vi "Sparse Signal FFT.vi"(2 "signal length":i32=1, 3 "X":cdb[](array[numeric]) format="%.2f") -> (0 "error":i32, 1 "FFT {X}":cdb[](array[numeric]) format="%.2f")   [LabVIEW 2020, in "NI_Gmath.lvlib"]
doc: "Computes the Fourier transform of sparse signals faster than the FFT does."
uses:
  <vilib>/gmath/NI_Gmath.lvlib
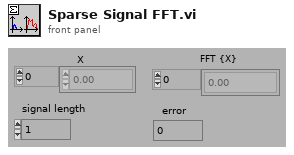
[diagram p1: front panel]
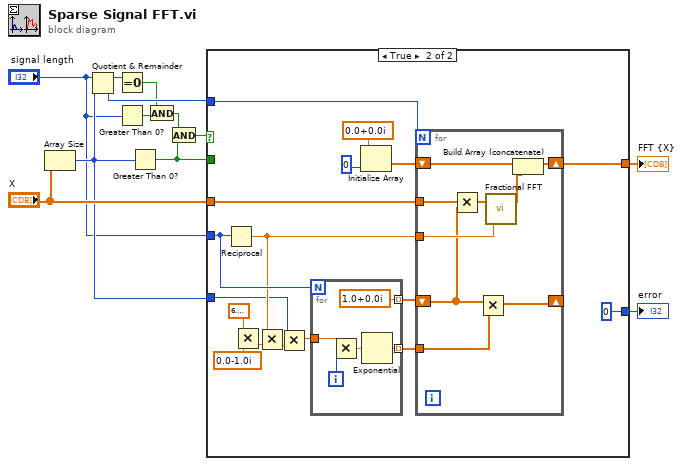
[diagram p0: block diagram]
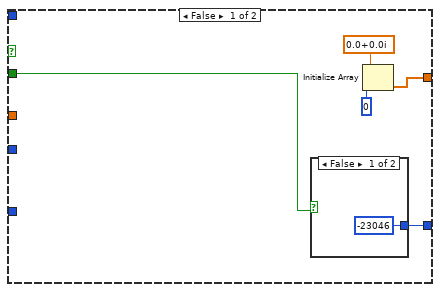
[diagram p2: hidden frame]
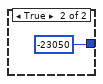
[diagram p3: hidden frame]
diagram:
  n1 = Array Size(array="X") -> (size(s)=w5:i32)
  n2 = Quotient & Remainder(x="signal length", y=w5) -> (x-y*floor(x/y)=w11:i32, floor(x/y)=w9:i32)
  n3 = Equal To 0?(x=w11) -> (x = 0?=w2:bool)
  n4 = Greater Than 0?(x="signal length") -> (x > 0?=w3:bool)
  n5 = Greater Than 0?(x=w5) -> (x > 0?=w8:bool)
  n6 = And(x=w2, y=w3) -> (x .and. y?=w1:bool)
  n7 = And(x=w1, y=w8) -> (x .and. y?=w10:bool)
  n8 = case shown="True" w10 {
    tunnel: "X" -> [_ w35]
    tunnel: [w15 w31] -> w7
    tunnel: [w13 0] -> w12
    tunnel: w8 -> [w14 _]
    tunnel: "signal length" -> [_ w25]
    tunnel: w9 -> [_ w21]
    tunnel: w5 -> [_ w20]
    frame False {
      n9 = case shown="False" w14 {
        tunnel: [-23046 -23050] -> w13
        frame False {
        }
        frame True {
        }
      }
      n10 = Initialize Array(cdb 0.0+0.0i, 0) -> (w15:cdb[])
    }
    frame True {
      n11 = Reciprocal(x=w25) -> (1/x=w24:dbl)
      n12 = Multiply(x=6.283185307179586, y=cdb 0.0-1.0i) -> (x*y=w28:cdb)
      n13 = Multiply(x=w24, y=w28) -> (x*y=w22:cdb)
      n14 = Multiply(x=w20, y=w22) -> (x*y=w23:cdb)
      n15 = for {
        N: w25 -> [_]
        tunnel: w23 -> [w41]
        tunnel: [w38] -> w27 mode=indexing
        tunnel: [cdb 1.0+0.0i] -> w26 mode=indexing
        i -> [w40]
        n16 = Multiply(x=w41, y=w40) -> (x*y=w39:cdb)
        n17 = Exponential(1:w39) -> (0:w38:cdb)
      }
      n18 = Initialize Array(cdb 0.0+0.0i, 0) -> (w32:cdb[])
      n19 = for {
        N: w21 -> [_]
        tunnel: w35 -> [w46]
        tunnel: w24 -> [w50]
        shift-right: [w48] -> w31
        shift-left: w32 -> [w49]
        tunnel: w27 -> [w47]
        shift-right: [w43] -> _
        shift-left: w26 -> [w42]
        n20 = Multiply(x=w46, y=w42) -> (x*y=w45:cdb[])
        n21 = Multiply(x=w42, y=w47) -> (x*y=w43:cdb[])
        n22 = call <vilib>:"Fractional FFT.vi"("alpha"=w50, "X"=w45) -> ("Fract FFT {X}"=w44:cdb[])  [unwired: 1 out]
        n23 = Build Array (concatenate)(w49, w44) -> (w48:cdb[])
      }
    }
  }
  "FFT {X}" <- w7
  "error" <- w12
